vi "Read Minor Frames.vi"(8 "error in":errorcluster, 11 "channel ref in":refnum<k20>) -> (0 "error out":errorcluster, 1 "minor frame period (us)":i32, 2 "minor frames":T1[](array[typedef]), 3 "channel ref out":refnum<k20>)   [LabVIEW 2020, in "MIL-STD 1553 Import.lvlib"]
uses:
  MIL-STD 1553 Import.lvlib
  Shared/Minor Frame Definition.ctl
  a26b07f3-20e1-4114-9005-43d73faf7b48.vi
  a26b07f3-20e1-4114-9005-43d73faf7b48.vi/b1e6fcf8-dac1-42d2-b1fe-151afe06dbd4.vi
  93a80e05-2db4-4bd5-86da-32f29481b94b.vi/b1e6fcf8-dac1-42d2-b1fe-151afe06dbd4.vi
  93a80e05-2db4-4bd5-86da-32f29481b94b.vi/b1e6fcf8-dac1-42d2-b1fe-151afe06dbd4.vi/bff94617-1577-41e8-ae99-0a9b0a2fdf5b.vi
  Constants.vi
  <vilib>/Utility/error.llb/Error Cluster From Error Code.vi
  <vilib>/xml/NI_XML.lvlib
  8eca2d5f-955d-43c4-8be7-97fb462d4491.vi
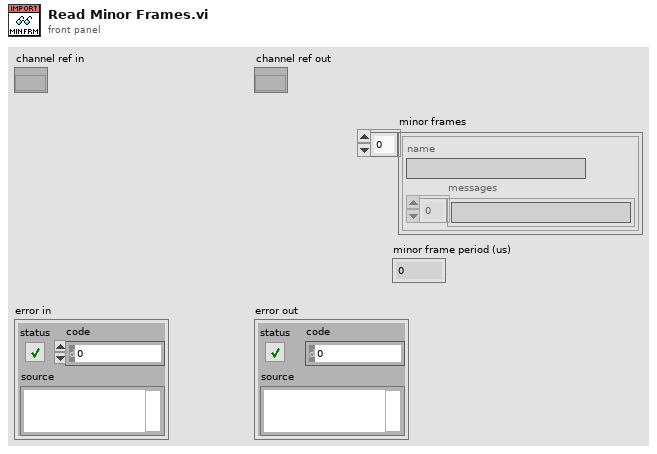
[diagram p1: front panel]
types:
  T1 = typedef "Minor Frame Definition.ctl" = cluster{"name":string, "messages":string[]}
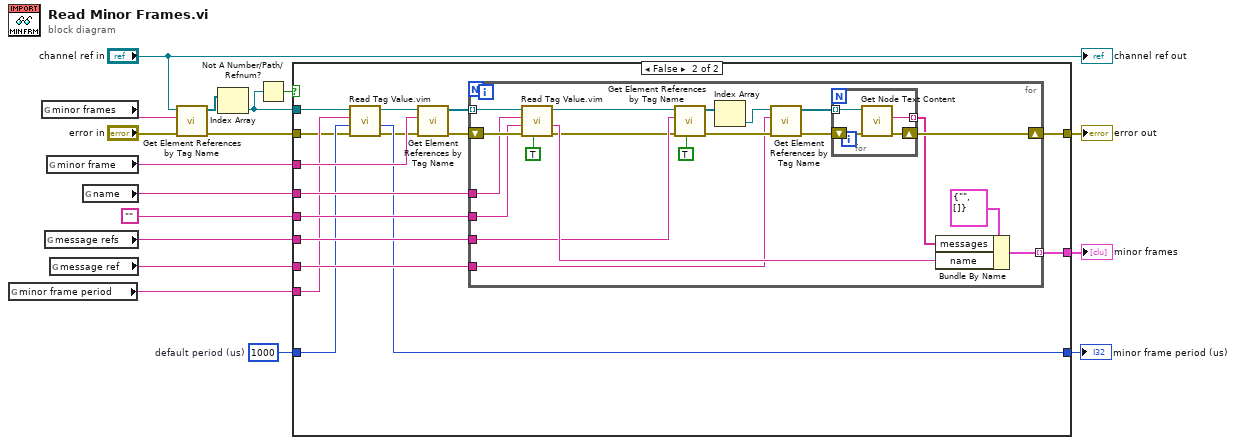
[diagram p0: block diagram]
diagram:
  w1 = 1000  # default period (us)
  n1 = global read "Constants.vi" "minor frame period"() -> (w3:string)
  n2 = global read "Constants.vi" "minor frames"() -> (w8:string)
  n3 = global read "Constants.vi" "message refs"() -> (w5:string)
  n4 = global read "Constants.vi" "minor frame"() -> (w17:string)
  n5 = global read "Constants.vi" "message ref"() -> (w4:string)
  n6 = global read "Constants.vi" "name"() -> (w15:string)
  n7 = call "Get Element References by Tag Name.vi"("error in"="error in", "tag name"=w8, "node in"="channel ref in") -> ("error out"=w10:errorcluster, "array of elements"=w12:refnum<k20>[])  [unwired: 7 in]
  n8 = Index Array(array=w12) -> (element=w9:refnum<k20>)  [unwired: 1 in]
  n9 = Not A Number/Path/Refnum?(number/path/refnum=w9) -> (NaN/Path/Refnum?=w6:bool)
  n10 = case shown="False" w6 {
    tunnel: w17 -> [_ w35]
    tunnel: [w19 w33] -> w16
    tunnel: w15 -> [_ w31]
    tunnel: "" -> [_ w30]
    tunnel: [_ w29] -> w13
    tunnel: w10 -> [w19 w23]
    tunnel: w9 -> [_ w20]
    tunnel: w5 -> [_ w28]
    tunnel: w4 -> [_ w27]
    tunnel: w3 -> [_ w26]
    tunnel: [w18 w25] -> w2
    tunnel: w1 -> [w18 w24]
    frame True {
    }
    frame False {
      n11 = call "Read Tag Value.vim"("error in"=w23, "default"=w24, "tag name"=w26, "node in"=w20) -> ("error out"=w22:errorcluster, "value"=w25:i32, "node out"=w21:refnum<k20>)  [unwired: 5 in]
      n12 = call "Get Element References by Tag Name.vi"("error in"=w22, "tag name"=w35, "node in"=w21) -> ("error out"=w32:errorcluster, "array of elements"=w34:refnum<k20>[])  [unwired: 7 in]
      n13 = for {
        shift-right: [w39] -> w33
        shift-left: w32 -> [w55]
        tunnel: w34 -> [w54] mode=indexing
        tunnel: w31 -> [w53]
        tunnel: w30 -> [w52]
        tunnel: [w49] -> w29 mode=indexing
        tunnel: w28 -> [w46]
        tunnel: w27 -> [w42]
        n14 = call "Read Tag Value.vim"("required (F)"=TRUE, "error in"=w55, "default"=w52, "tag name"=w53, "node in"=w54) -> ("error out"=w37:errorcluster, "value"=w50:string, "node out"=w36:refnum<k20>)  [unwired: 4 in]
        n15 = call "Get Element References by Tag Name.vi"("required (F)"=TRUE, "error in"=w37, "tag name"=w46, "node in"=w36) -> ("error out"=w43:errorcluster, "array of elements"=w45:refnum<k20>[])  [unwired: 6 in]
        n16 = Index Array(array=w45) -> (element=w44:refnum<k20>)  [unwired: 1 in]
        n17 = call "Get Element References by Tag Name.vi"("error in"=w43, "tag name"=w42, "node in"=w44) -> ("error out"=w40:errorcluster, "array of elements"=w41:refnum<k20>[])  [unwired: 7 in]
        n18 = for {
          tunnel: w41 -> [w59] mode=indexing
          shift-right: [w57] -> w39
          shift-left: w40 -> [w58]
          tunnel: [w56] -> w38 mode=indexing
          n19 = call <vilib>:"Get Node Text Content.vi"("error in (no error)"=w58, "node in"=w59) -> ("error out"=w57:errorcluster, "node text"=w56:string)  [unwired: 7 in, 1 out]
        }
        n20 = Bundle By Name(cluster=T1 {"name"="", "messages"=[]} ("minor frame definition"), "messages"=w38, "name"=w50) -> (w49:T1)
      }
    }
  }
  "error out" <- w16
  "minor frames" <- w13
  "minor frame period (us)" <- w2
  "channel ref out" <- "channel ref in"
